vi "Add init and unlock.vi"(8 "error in (no error)":errorcluster, 10 "message in":string, 11 "ICS in":refnum<class "ICS.lvclass">) -> (0 "error out":errorcluster, 1 "unlock":bool, 2 "message out":string, 3 "ICS out":refnum<class "ICS.lvclass">)   [LabVIEW 2018, in "ICS.lvclass"]
uses:
  ICS.lvclass
  ICS.lvclass/ICS.ctl
  Motor/Motor.lvclass
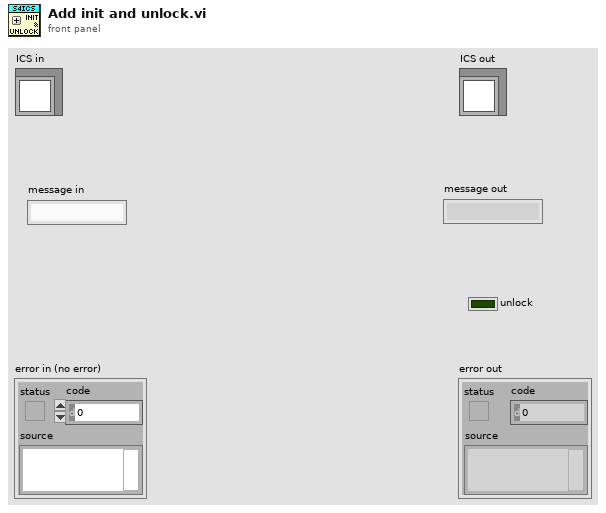
[diagram p1: front panel]
types:
  T1 = cluster{"action":string, "param":string, "pos_name":string, "pos_idx":i32, "ack":bool, "stop":bool, "offset":bool, "immediate":bool, "instructions":string[]}
  T2 = cluster{"mode":string, "condition":string, "position":string, "pos_name":string, "pos_id":string}
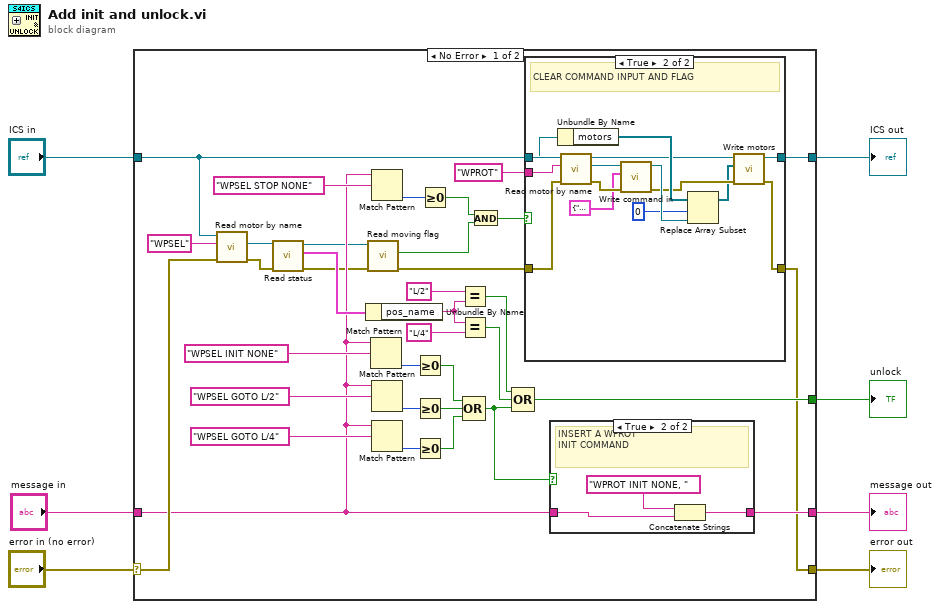
[diagram p0: block diagram]
diagram:
  n1 = case shown="No Error" "error in (no error)" {
    selector: "error in (no error)" -> [w41 w63]
    tunnel: [w14 w63] -> w6
    tunnel: [w16 w64] -> w4
    tunnel: "ICS in" -> [w17 w64]
    tunnel: [w22 _] -> w3
    tunnel: "message in" -> [w18 _]
    tunnel: [w21 _] -> w1
    frame No Error {
      n2 = call-dynamic "Read motor by name.vi"("error in (no error)"=w41, "motor name"="WPSEL", "ICS in"=w17) -> ("error out"=w39:errorcluster, "Motor.lvclass"=w40:refnum<class "Motor.lvclass">)  [unwired: 5 in, 2 out]
      n3 = call-dynamic "Read status.vi"("error in (no error)"=w39, "Motor in"=w40) -> ("error out"=w13:errorcluster, "status"=w38:T2, "Motor out"=w11:refnum<class "Motor.lvclass">)  [unwired: 6 in, 1 out]
      n4 = Unbundle By Name(w38) -> ("pos_name"=w37:string)
      n5 = call-dynamic "Read moving flag.vi"("error in (no error)"=w13, "Motor in"=w11) -> ("error out"=w12:errorcluster, "moving"=w10:bool)  [unwired: 7 in, 1 out]
      n6 = Match Pattern(string=w18, regular expression="WPSEL INIT NONE") -> (offset past match=w29:i32)  [unwired: 1 in, 3 out]
      n7 = Match Pattern(string=w18, regular expression="WPSEL STOP NONE") -> (offset past match=w19:i32)  [unwired: 1 in, 3 out]
      n8 = Match Pattern(string=w18, regular expression="WPSEL GOTO L/2") -> (offset past match=w30:i32)  [unwired: 1 in, 3 out]
      n9 = Match Pattern(string=w18, regular expression="WPSEL GOTO L/4") -> (offset past match=w31:i32)  [unwired: 1 in, 3 out]
      n10 = Greater Or Equal To 0?(x=w29) -> (x >= 0?=w32:bool)
      n11 = Greater Or Equal To 0?(x=w30) -> (x >= 0?=w33:bool)
      n12 = Greater Or Equal To 0?(x=w31) -> (x >= 0?=w34:bool)
      n13 = Greater Or Equal To 0?(x=w19) -> (x >= 0?=w9:bool)
      n14 = Equal?(x="L/2" ("motor name"), y=w37) -> (x = y?=w25:bool)
      n15 = Equal?(x=w37, y="L/4" ("motor name")) -> (x = y?=w24:bool)
      n16 = Compound Arithmetic op=OR(w32, w33, w34) -> (w23:bool)
      n17 = And(x=w9, y=w10) -> (x .and. y?=w8:bool)
      n18 = Compound Arithmetic op=OR(w25, w24, w23) -> (w22:bool)
      n19 = case shown="True" w8 {
        tunnel: w17 -> [w44 w58]
        tunnel: [w44 w49] -> w16
        tunnel: w12 -> [w43 w57]
        tunnel: "WPROT" ("motor name") -> [_ w56]
        tunnel: [w43 w46] -> w14
        frame False {
        }
        frame True {
          # "CLEAR COMMAND INPUT AND FLAG"
          n20 = call-dynamic "Read motor by name.vi"("error in (no error)"=w57, "motor name"=w56, "ICS in"=w58) -> ("error out"=w54:errorcluster, "Motor.lvclass"=w55:refnum<class "Motor.lvclass">, "ICS out"=w50:refnum<class "ICS.lvclass">)  [unwired: 5 in, 1 out]
          n21 = Unbundle By Name(w50) -> ("motors"=w53:refnum<class "Motor.lvclass">[])
          n22 = call-dynamic "Write command in.vi"("error in (no error)"=w54, "command in"=T1 {"action"="", "param"="", "pos_name"="", "pos_idx"=0, "ack"=FALSE, "stop"=FALSE, "offset"=FALSE, "immediate"=FALSE, "instructions"=[]}, "Motor in"=w55) -> ("error out"=w48:errorcluster, "Motor out"=w52:refnum<class "Motor.lvclass">)  [unwired: 7 in]
          n23 = Replace Array Subset(array=w53, new element=w52, index=0) -> (w47:refnum<class "Motor.lvclass">[])
          n24 = call-dynamic "Write motors.vi"("error in (no error)"=w48, "motors"=w47, "ICS in"=w50) -> ("error out"=w46:errorcluster, "ICS out"=w49:refnum<class "ICS.lvclass">)  [unwired: 7 in]
        }
      }
      n25 = case shown="True" w23 {
        tunnel: w18 -> [w59 w61]
        tunnel: [w59 w62] -> w21
        frame False {
          # "NO WPSEL COMMAND THAT  \nREQUIRES WPROT INIT"
        }
        frame True {
          # "INSERT A WPROT \nINIT COMMAND"
          n26 = Concatenate Strings("WPROT INIT NONE, " ("regular expression"), w61) -> (w62:string)
        }
      }
    }
    frame Error {
    }
  }
  "error out" <- w6
  "ICS out" <- w4
  "unlock" <- w3
  "message out" <- w1
